vi "Intan_SetStreamChans.vi"(0 "Amplifier Chans":i32[](listbox)=[1, 4, 13, 14, 15, 16, 17, 22], 1 "Accel/Vbat":i32[](listbox)) -> (2 "ChanSelect(uint32)":u32[](array[numeric]), 3 "ChanSelString":string, 4 "BitMaskAll":bool[](array[boolean]))   [LabVIEW 2020]
doc: "Takes in listbox of channels to stream (amps A-D, ADXL+Vbat) and generates the 5x uint32 numbers to set which channels to stream on Intsy.\n1st number: Amp A chans\n2nd number: Amp B chans\n3rd number: Amp C chans\n4th number: Amp D chans\n5th number: (ax,ay,az, Vbat)"
panel:
  out "uint32num":u32
  out "sub bitmask":bool[](array[boolean])
  out "AdxlVddOn":i16[](array[numeric])
  out "AmpOnIndx":i16[](array[numeric])
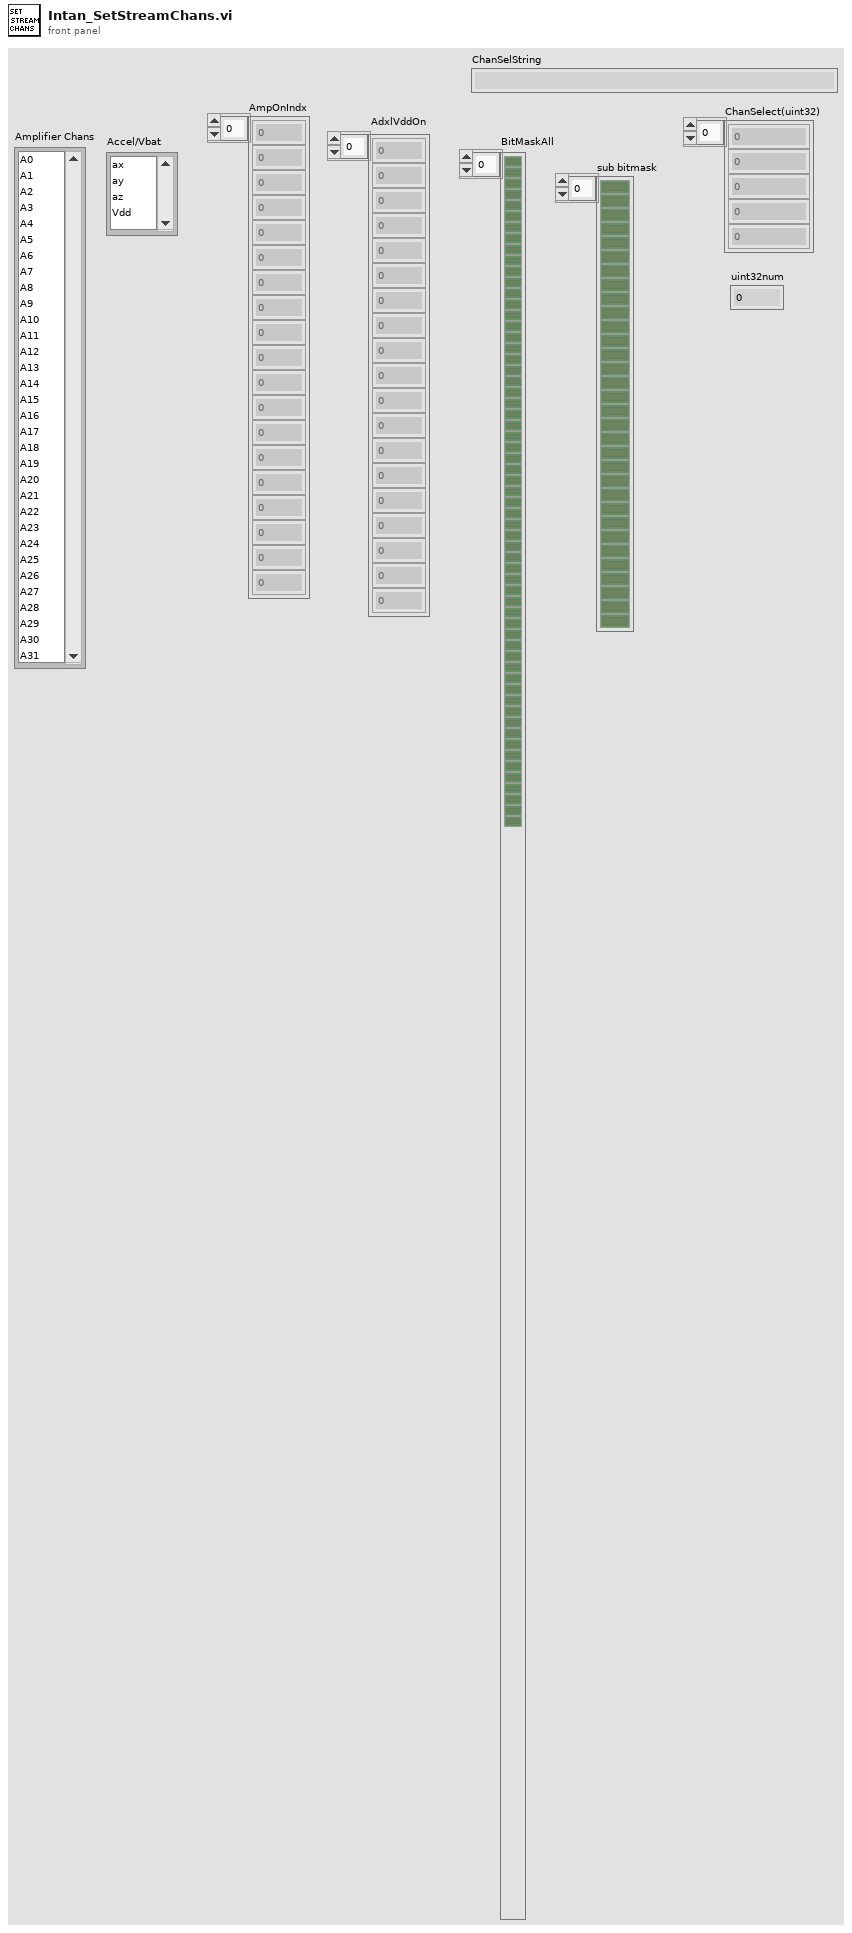
[diagram p1: front panel]
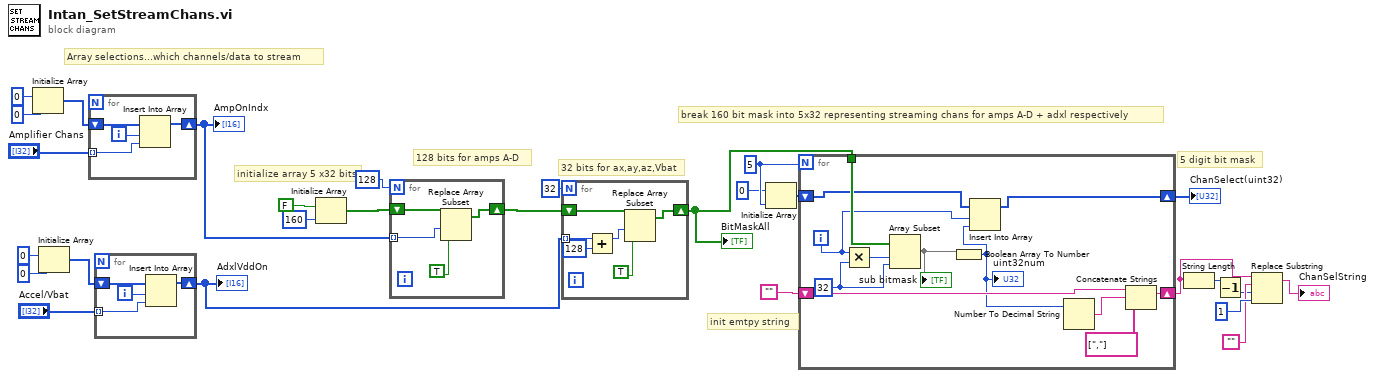
[diagram p0: block diagram]
diagram:
  w11 = 5
  # "init emtpy string"
  # "break 160 bit mask into 5x32 representing streaming chans for amps A-D + adxl respectively"
  # "5 digit bit mask"
  # "Array selections...which channels/data to stream"
  # "32 bits for ax,ay,az,Vbat"
  # "128 bits for amps A-D"
  # "initialize array 5 x32 bits"
  n1 = Initialize Array(i16 0 ("element"), 0 ("dimension size")) -> (w26:i16[])
  n2 = Initialize Array(i16 0 ("element"), 0 ("dimension size")) -> (w23:i16[])
  n3 = for {
    tunnel: "Amplifier Chans" -> [w31] mode=indexing
    shift-right: [w29] -> w20
    shift-left: w26 -> [w32]
    i -> [w30]
    n4 = Insert Into Array(array=w32, index=w30, new element=w31) -> (w29:i16[])
  }
  "AmpOnIndx" <- w20
  n5 = for {
    tunnel: "Accel/Vbat" -> [w35] mode=indexing
    shift-right: [w33] -> w13
    shift-left: w23 -> [w36]
    i -> [w34]
    n6 = Insert Into Array(array=w36, index=w34, new element=w35) -> (w33:i16[])
  }
  "AdxlVddOn" <- w13
  n7 = Initialize Array(FALSE ("Boolean"), 160 ("dimension size")) -> (w16:bool[])
  n8 = for {
    N: 128 ("dimension size") -> [_]
    tunnel: w20 -> [w38] mode=indexing
    shift-right: [w39] -> w14
    shift-left: w16 -> [w40]
    n9 = Replace Array Subset(array=w40, new element=TRUE ("new element/subarray"), index=w38) -> (w39:bool[])
  }
  n10 = for {
    N: 32 -> [_]
    tunnel: w13 -> [w44] mode=indexing
    shift-right: [w45] -> w12
    shift-left: w14 -> [w46]
    n11 = Add(x=w44, y=i16 128) -> (x+y=w42:i16)
    n12 = Replace Array Subset(array=w46, new element=TRUE ("new element/subarray"), index=w42) -> (w45:bool[])
  }
  "BitMaskAll" <- w12
  n13 = Initialize Array(u32 0 ("dimension size"), w11) -> (w9:u32[])
  n14 = for {
    N: w11 -> [_]
    tunnel: w12 -> [w58]
    shift-right: [w52] -> w8
    shift-left: w9 -> [w54]
    shift-right: [w50] -> w6
    shift-left: "" -> [w49]
    i -> [w53]
    w56 = 32 ("length")
    n15 = Multiply(x=w53, y=w56) -> (x*y=w57:i32)
    n16 = Array Subset(array=w58, index=w57, length=w56) -> (w55:bool[])
    "sub bitmask" <- w55
    n17 = Boolean Array To Number(Boolean array=w55) -> (number=w47:u32)
    "uint32num" <- w47
    n18 = Insert Into Array(array=w54, index=w53, new element=w47) -> (w52:u32[])
    n19 = Number To Decimal String(number=w47) -> (decimal integer string=w51:string)  [unwired: 1 in]
    n20 = Concatenate Strings(w49, w51, string[] [","] ("string")) -> (w50:string)
  }
  "ChanSelect(uint32)" <- w8
  n21 = String Length(string=w6) -> (length=w5:i32)
  n22 = Decrement(x=w5) -> (x-1=w1:i32)
  n23 = Replace Substring(2:1 ("length (len. of substring)"), 3:w1, 4:"", 5:w6) -> (1:→"ChanSelString":string)  [unwired: 1 out]
